vi "All Child Values.vi"(11 "Long Class Name Entity Example in":refnum<class "Long Class Name Entity Example.lvclass">) -> (2 "All Values":refnum<class "Type.lvclass">[](array[class]))   [LabVIEW 2022 SP3, in "Conditum-Example.lvlib" / "Long Class Name Entity Example.lvclass"]
uses:
  Long Class Name Entity Example.lvclass
  Conditum/Columns/Type/Type.lvclass
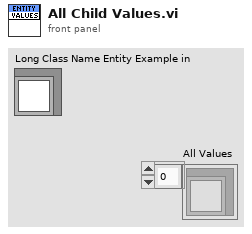
[diagram p1: front panel]
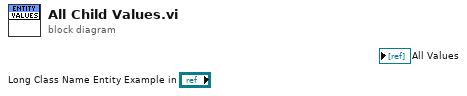
[diagram p0: block diagram]
diagram:
